vi "FPGA_EncoderERRInvalidResource.vi"(1 "error in (no error)":errorcluster) -> (0 "error out":errorcluster={"status"=TRUE, "code"=1, "source"="Invalid Encoder Index Error."})   [LabVIEW 2017]
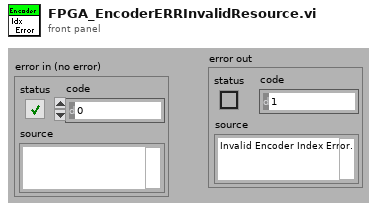
[diagram p1: front panel]
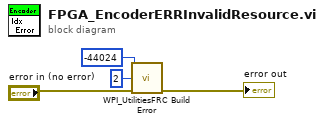
[diagram p0: block diagram]
diagram:
  n1 = call <vilib>:"WPI_UtilitiesFRC Build Error.vi"("error code"=-44024 ("code"), "chain levels to remove (1)"=2, "error in (no error)"="error in (no error)") -> ("error out"=→"error out":errorcluster)  [unwired: 2 in, 10 out]
